vi "Execute AT command.vi"(5 "Exit AT mode":bool, 6 "milliseconds to wait":u32=100, 7 "error in (no error)":errorcluster, 8 "AT Command":string, 10 "VISA resource in":refnum<visa-resource-name>) -> (0 "error out":errorcluster, 2 "Response message":string, 3 "VISA resource out":refnum<visa-resource-name>)   [LabVIEW 2017]
uses:
  <vilib>/Instr/_visa.llb/VISA Flush IO Buffer Mask.ctl
  Mode enum.ctl
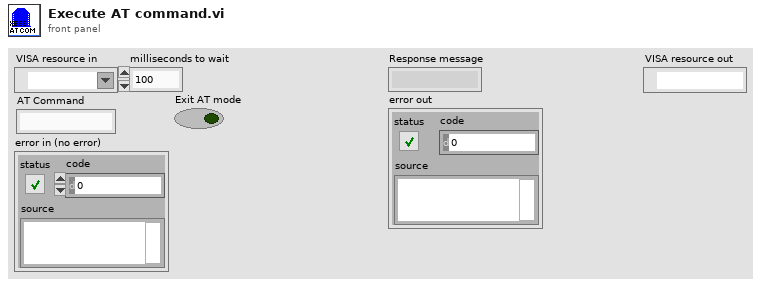
[diagram p1: front panel]
types:
  T1 = typedef "Mode enum.ctl" = enum16{"Other", "Command mode"}
  T2 = typedef "VISA Flush IO Buffer Mask.ctl" = u16
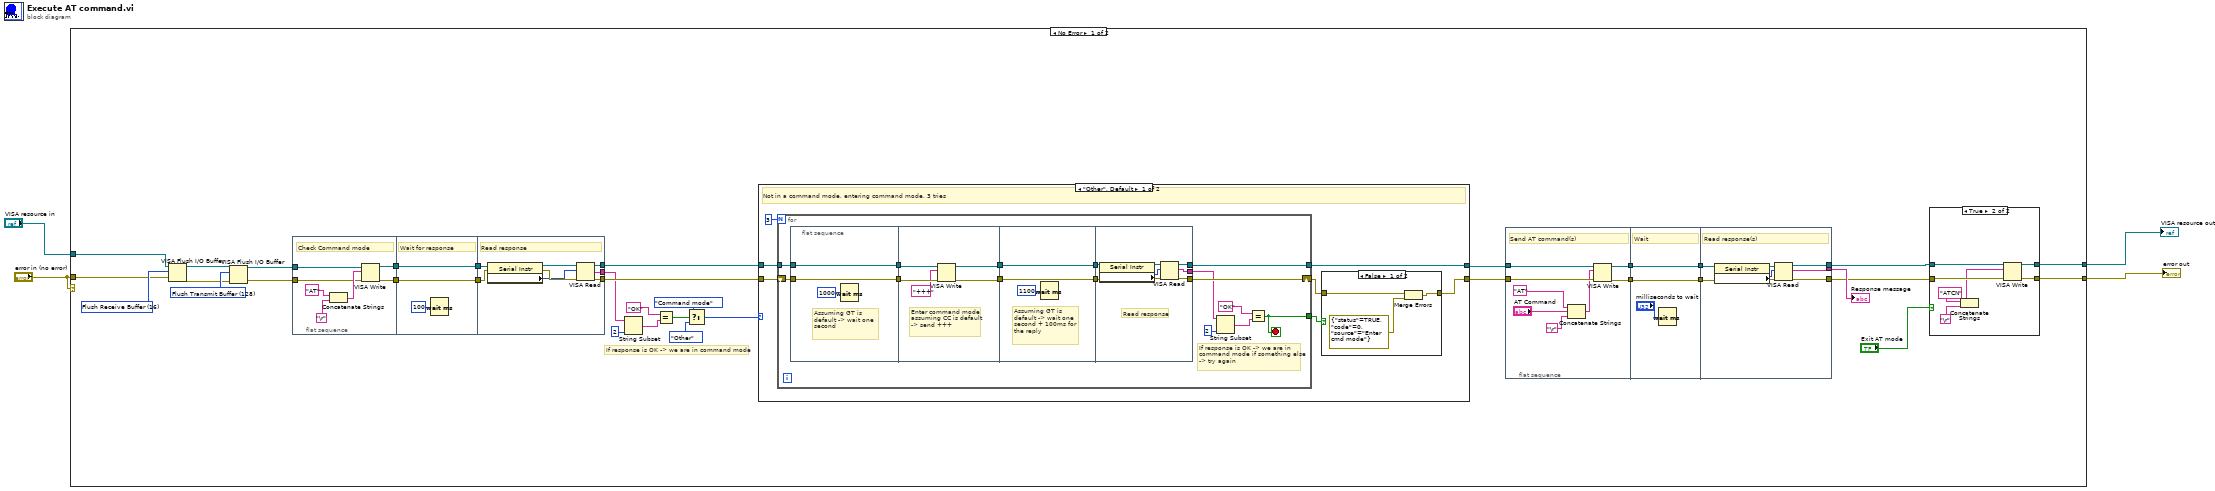
[diagram p0: block diagram]
diagram:
  n1 = case shown="No Error" "error in (no error)" {
    tunnel: "VISA resource in" -> [w24 w132]
    tunnel: "error in (no error)" -> [w17 w133]
    tunnel: [w13 w132] -> w3
    tunnel: [w12 w133] -> w2
    frame No Error {
      w25 = T2 16 items=["Flush Receive Buffer"=16, "Write Transmit Buffer to Device"=32, "Flush Receive Buffer (No I/O)"=64, "Flush Transmit Buffer"=128] ("Mask")
      w30 = T2 128 items=["Flush Receive Buffer"=16, "Write Transmit Buffer to Device"=32, "Flush Receive Buffer (No I/O)"=64, "Flush Transmit Buffer"=128] ("Mask")
      # "If response is OK -> we are in command mode"
      n2 = VISA Flush I/O Buffer(VISA resource name=w24, mask (16)=w25, error in (no error)=w17) -> (VISA resource name out=w27:refnum<visa-resource-name>, error out=w26:errorcluster)
      n3 = VISA Flush I/O Buffer(VISA resource name=w27, mask (16)=w30, error in (no error)=w26) -> (VISA resource name out=w29:refnum<visa-resource-name>, error out=w28:errorcluster)
      n4 = flat-sequence {
        tunnel: w29 -> [w45]
        tunnel: w28 -> [w42]
        tunnel: [w40] -> w34
        tunnel: [w39] -> w33
        tunnel: w34 -> [w47]
        tunnel: w33 -> [w46]
        tunnel: [w47] -> w32
        tunnel: [w46] -> w31
        tunnel: w32 -> [w56]
        tunnel: w31 -> [w55]
        tunnel: [w51] -> w22
        tunnel: [w50] -> w21
        tunnel: [w49] -> w11
        frame #0 {
          # "Check Command mode"
          n5 = Concatenate Strings("AT" ("string"), "\r") -> (w43:string)
          n6 = VISA Write(VISA resource name=w45, write buffer=w43, error in (no error)=w42) -> (VISA resource name out=w40:refnum<visa-resource-name>, error out=w39:errorcluster)  [unwired: 1 out]
        }
        frame #1 {
          # "Wait for response"
          n7 = Wait (ms)(milliseconds to wait=u32 100 ("millisecond multiple")) -> ()  [unwired: 1 out]
        }
        frame #2 {
          # "Read response"
          n8 = property class="Serial Instr"(reference=w56, error in=w55) -> (reference out=w54:refnum<visa-resource-name>, error out=w53:errorcluster, "Serial Settings:Number of Bytes at Serial Port"=w52:u32)
          n9 = VISA Read(VISA resource name=w54, byte count=w52, error in (no error)=w53) -> (VISA resource name out=w51:refnum<visa-resource-name>, read buffer=w49:string, error out=w50:errorcluster)  [unwired: 1 out]
        }
      }
      n10 = String Subset(string=w11, length (rest)=2 ("length (rest)")) -> (substring=w9:string)  [unwired: 1 in]
      n11 = Equal?(x="OK", y=w9) -> (x = y?=w7:bool)
      n12 = Select(t=Mode_enum."Command mode", s=w7, f=Mode_enum."Other") -> (s? t:f=w23:T1)
      n13 = case shown="\"Other\", Default" w23 {
        tunnel: w22 -> [w91 w131]
        tunnel: w21 -> [w90 w130]
        tunnel: [w89 w131] -> w20
        tunnel: [w85 w130] -> w19
        frame "Other", Default {
          # "Not in a command mode, entering command mode, 3 tries"
          n14 = for {
            N: 3 -> [_]
            shift-right: [w101] -> w86
            shift-left: w90 -> [w103]
            tunnel: w91 -> [w104]
            tunnel: [w102] -> w89
            tunnel: [w96] -> w87
            stop <- w96 stop-if-true
            # "If response is OK -> we are in command mode if something else -> try again"
            n15 = flat-sequence {
              tunnel: w104 -> [w112]
              tunnel: w103 -> [w111]
              tunnel: [w112] -> w110
              tunnel: [w111] -> w109
              tunnel: w110 -> [w118]
              tunnel: w109 -> [w117]
              tunnel: [w116] -> w108
              tunnel: [w115] -> w107
              tunnel: w108 -> [w121]
              tunnel: w107 -> [w120]
              tunnel: [w121] -> w106
              tunnel: [w120] -> w105
              tunnel: [w123] -> w101
              tunnel: [w124] -> w102
              tunnel: w106 -> [w129]
              tunnel: w105 -> [w128]
              tunnel: [w122] -> w97
              frame #0 {
                # "Assuming GT is default -> wait one second"
                n16 = Wait (ms)(milliseconds to wait=u32 1000) -> ()  [unwired: 1 out]
              }
              frame #1 {
                # "Enter command mode assuming CC is default -> send +++"
                n17 = VISA Write(VISA resource name=w118, write buffer="+++", error in (no error)=w117) -> (VISA resource name out=w116:refnum<visa-resource-name>, error out=w115:errorcluster)  [unwired: 1 out]
              }
              frame #2 {
                # "Assuming GT is default -> wait one second + 100ms for the reply"
                n18 = Wait (ms)(milliseconds to wait=u32 1100) -> ()  [unwired: 1 out]
              }
              frame #3 {
                # "Read response"
                n19 = property class="Serial Instr"(reference=w129, error in=w128) -> (reference out=w125:refnum<visa-resource-name>, error out=w127:errorcluster, "Serial Settings:Number of Bytes at Serial Port"=w126:u32)
                n20 = VISA Read(VISA resource name=w125, byte count=w126, error in (no error)=w127) -> (VISA resource name out=w124:refnum<visa-resource-name>, read buffer=w122:string, error out=w123:errorcluster)  [unwired: 1 out]
              }
            }
            n21 = String Subset(string=w97, length (rest)=2 ("length (rest)")) -> (substring=w99:string)  [unwired: 1 in]
            n22 = Equal?(x="OK", y=w99) -> (x = y?=w96:bool)
          }
          n23 = case shown="False" w87 {
            tunnel: w86 -> [w93 w95]
            tunnel: [w94 w95] -> w85
            frame False {
              n24 = Merge Errors(w93, errorcluster {"status"=TRUE, "code"=0, "source"="Enter cmd mode"} ("error constant")) -> (w94:errorcluster)
            }
            frame True {
            }
          }
        }
        frame "Command mode" {
          # "In command mode, no action required"
        }
      }
      n25 = flat-sequence {
        tunnel: w20 -> [w73]
        tunnel: w19 -> [w72]
        tunnel: [w67] -> w38
        tunnel: [w66] -> w37
        tunnel: w38 -> [w76]
        tunnel: w37 -> [w75]
        tunnel: [w76] -> w36
        tunnel: [w75] -> w35
        tunnel: w36 -> [w84]
        tunnel: w35 -> [w83]
        tunnel: [w79] -> w18
        tunnel: [w78] -> w14
        tunnel: [w77] -> w15
        frame #0 {
          # "Send AT command(s)"
          n26 = Concatenate Strings("AT" ("string"), "AT Command", "\r") -> (w71:string)
          n27 = VISA Write(VISA resource name=w73, write buffer=w71, error in (no error)=w72) -> (VISA resource name out=w67:refnum<visa-resource-name>, error out=w66:errorcluster)  [unwired: 1 out]
        }
        frame #1 {
          # "Wait"
          n28 = Wait (ms)(milliseconds to wait="milliseconds to wait") -> ()  [unwired: 1 out]
        }
        frame #2 {
          # "Read response(s)"
          n29 = property class="Serial Instr"(reference=w84, error in=w83) -> (reference out=w80:refnum<visa-resource-name>, error out=w82:errorcluster, "Serial Settings:Number of Bytes at Serial Port"=w81:u32)
          n30 = VISA Read(VISA resource name=w80, byte count=w81, error in (no error)=w82) -> (VISA resource name out=w77:refnum<visa-resource-name>, read buffer=w79:string, error out=w78:errorcluster)  [unwired: 1 out]
        }
      }
      n31 = case shown="True" "Exit AT mode" {
        tunnel: w15 -> [w58 w65]
        tunnel: w14 -> [w57 w64]
        tunnel: [w58 w60] -> w13
        tunnel: [w57 w59] -> w12
        frame False {
        }
        frame True {
          n32 = Concatenate Strings("ATCN" ("write buffer"), "\r") -> (w62:string)
          n33 = VISA Write(VISA resource name=w65, write buffer=w62, error in (no error)=w64) -> (VISA resource name out=w60:refnum<visa-resource-name>, error out=w59:errorcluster)  [unwired: 1 out]
        }
      }
      "Response message" <- w18
    }
    frame Error {
    }
  }
  "VISA resource out" <- w3
  "error out" <- w2
